vi "ui get log info.vi"(11 "txt file path":path) -> (1 "Destination":path[](array[path]), 3 "Source":path[](array[path]))   [LabVIEW 2023]
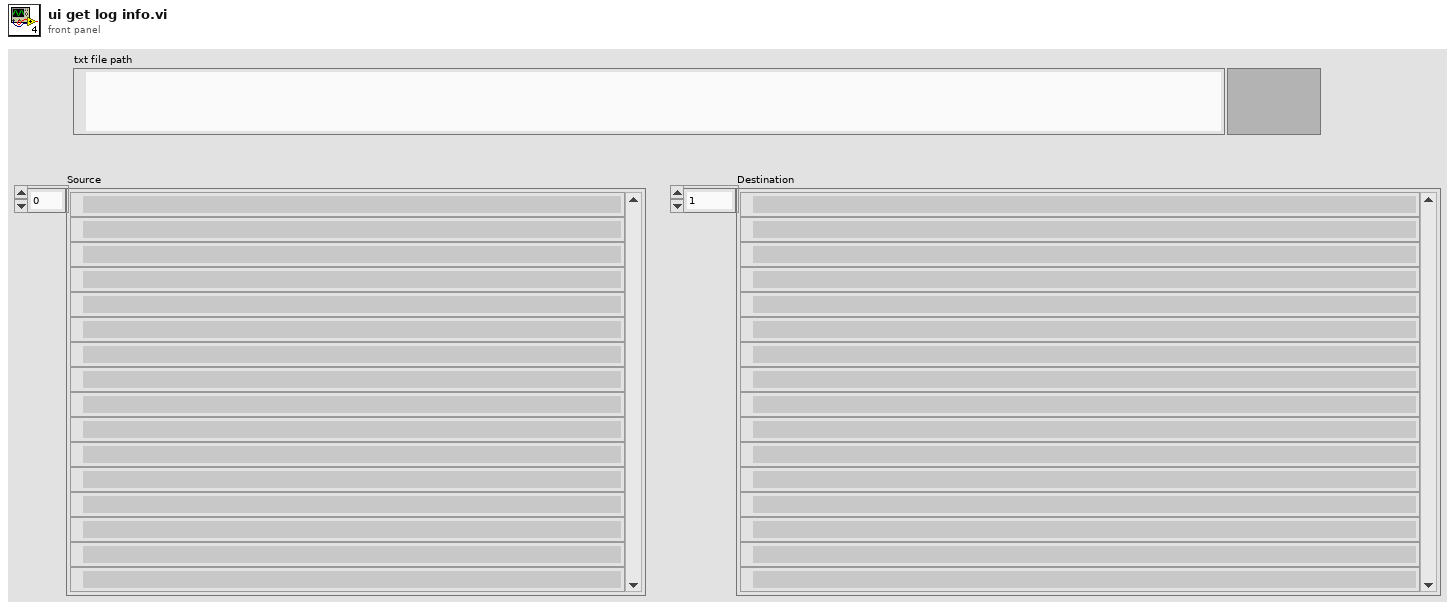
[diagram p1: front panel]
types:
  T1 = enum16{"Copying", "Moving", "Deleting", "Skiped", "Renaming"}
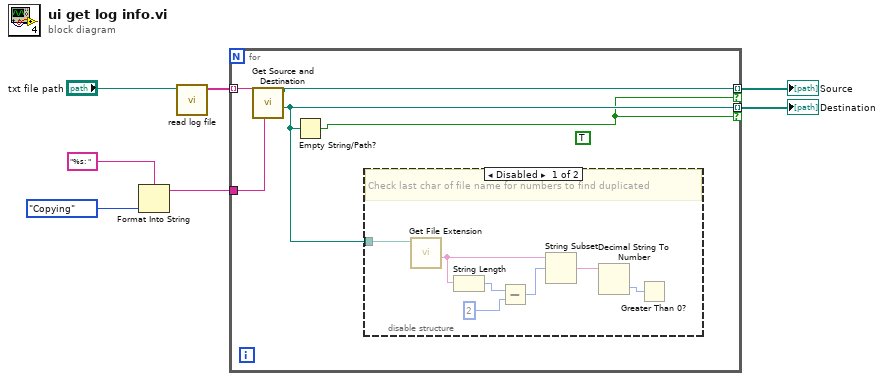
[diagram p0: block diagram]
diagram:
  n1 = Format Into String(format string="%s: ", T1."Copying" ("Operation")) -> (resulting string=w1:string)  [unwired: 2 in, 1 out]
  n2 = call "read log file.vi"("file (use dialog)"="txt file path") -> ("array"=w7:string[])  [unwired: 10 in]
  n3 = for {
    tunnel: w7 -> [w12] mode=indexing
    tunnel: [w11] -> w6 mode=indexing if=w8
    tunnel: [w10] -> w5 mode=indexing if=w8
    tunnel: w1 -> [w9]
    (unwired) TRUE
    n4 = call "Get Source and Destination.vi"("regular expression"=w9, "parh"=w12) -> ("Destination"=w10:path, "Source"=w11:path)  [unwired: 8 in]
    n5 = Empty String/Path?(string/path=w10) -> (empty?=w8:bool)
    n6 = disable-structure shown="Disabled" {
      disable-tunnel: w10 -> [w19 _]
      frame Disabled {
        # "Check last char of file name for numbers to find duplicated"
        n7 = call <vilib>:"Get File Extension.vi"("file"=w19) -> ("filename without extension"=w18:string)  [unwired: 6 in, 4 out]
        n8 = String Length(string=w18) -> (length=w17:i32)
        n9 = Subtract(x=w17, y=2) -> (x-y=w15:i32)
        n10 = String Subset(string=w18, offset (0)=w15) -> (substring=w14:string)  [unwired: 1 in]
        n11 = Decimal String To Number(string=w14) -> (number=w13:i32)  [unwired: 2 in, 1 out]
        n12 = Greater Than 0?(x=w13) -> ()  [unwired: 1 out]
      }
      frame Enabled {
      }
    }
  }
  "Source" <- w6
  "Destination" <- w5
